vi "SetMultipleConnectionScope.vi"(9 "Number of Connections size":i32=8, 10 "port or service name":u16, 11 "Remote Host":string) -> ()   [LabVIEW 2013]
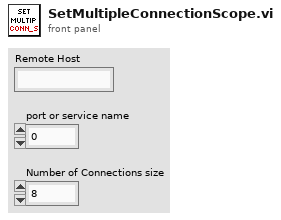
[diagram p1: front panel]
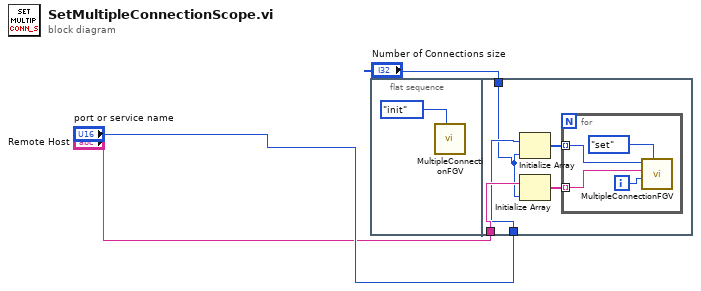
[diagram p0: block diagram]
diagram:
  n1 = flat-sequence {
    tunnel: "Remote Host" -> [w9]
    tunnel: "port or service name" -> [w7]
    tunnel: "Number of Connections size" -> [w5]
    frame #0 {
      n2 = call "MultipleConnectionFGV.vi"("command"=enum16{"get", "set", "init"}."init") -> ()  [unwired: 9 in, 2 out]
    }
    frame #1 {
      n3 = Initialize Array(w7, w5) -> (w6:u16[])
      n4 = Initialize Array(w9, w5) -> (w8:string[])
      n5 = for {
        tunnel: w6 -> [w12] mode=indexing
        tunnel: w8 -> [w11] mode=indexing
        i -> [w10]
        n6 = call "MultipleConnectionFGV.vi"("command"=enum16{"get", "set", "init"}."set", "Nr."=w10, "Remote Host in"=w11, "port or service name in"=w12) -> ()  [unwired: 6 in, 2 out]
      }
    }
  }
